vi "Get GObj Unique Name.vi"(8 "error in":errorcluster, 11 "GObj Refnum":refnum<vi>) -> (0 "error out":errorcluster, 2 "found?":bool, 3 "unique name":string)   [LabVIEW 2010, in "NI_SE_Front Panel Layout.lvlib"]
uses:
  NI_SE_Front Panel Layout.lvlib
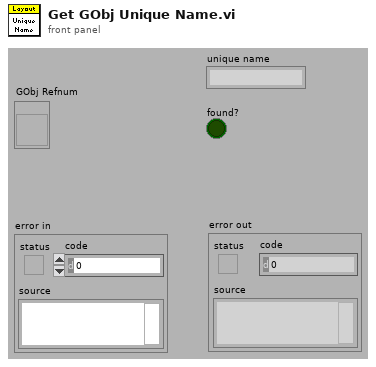
[diagram p1: front panel]
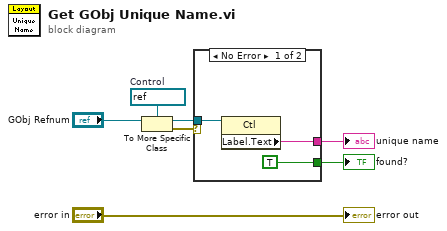
[diagram p0: block diagram]
diagram:
  w6 = refnum<vi> refnum  # Control
  n1 = To More Specific Class(target class=w6, reference="GObj Refnum") -> (specific class reference=w3:refnum<vi>, error out=w4:errorcluster)  [unwired: 1 in]
  n2 = case shown="No Error" w4 {
    tunnel: w3 -> [w10 _]
    tunnel: [w9 _] -> w2
    tunnel: [TRUE _] -> w1
    frame No Error {
      n3 = property class="Ctl"(reference=w10) -> ("Label.Text"=w9:string)  [unwired: 1 in, 2 out]
    }
    frame Error {
    }
  }
  "unique name" <- w2
  "found?" <- w1
  "error out" <- "error in"
